vi "Set Default Ref Phase.vi"(8 "error in (no error)":errorcluster, 10 "Default Phase Value (0.0 degrees)":dbl format="%.4f", 11 "VISA resource name":refnum<visa-resource-name>) -> (0 "error out":errorcluster, 3 "VISA resource name out":refnum<visa-resource-name>)   [LabVIEW 2011, in "Fluke 5XXX Series Multicalibrators.lvlib"]
doc: "If two Calibrators are synchronized using 10 MHz IN/OUT, sets the power-up and reset default phase difference between the primary channel on the Calibrator relative to the sync pulse on the 10 MHz IN or OUT terminal.\n\nNote:\n\nThis VI is available only for instrument model 5520A."
uses:
  Fluke 5XXX Series Multicalibrators.lvlib
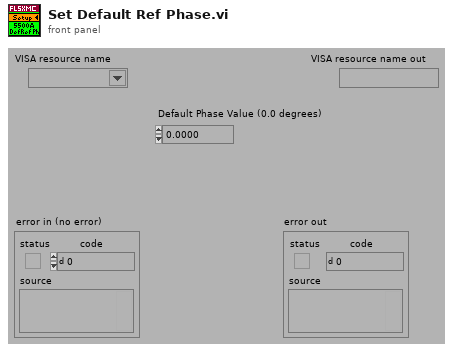
[diagram p1: front panel]
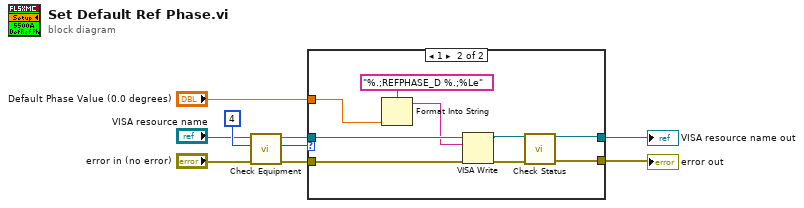
[diagram p0: block diagram]
diagram:
  n1 = call "Check Equipment.vi"("error in (no error)"="error in (no error)", "Bit Mask"=4 ("Numeric"), "VISA resource name"="VISA resource name") -> ("error out"=w9:errorcluster, "Present?"=w8:u32, "VISA resource name out"=w7:refnum<visa-resource-name>)  [unwired: 6 in]
  n2 = case shown="1" w8 {
    tunnel: "Default Phase Value (0.0 degrees)" -> [_ w12]
    tunnel: [w10 w15] -> w1
    tunnel: w9 -> [w11 w20]
    tunnel: w7 -> [w10 w19]
    tunnel: [w11 w18] -> w2
    frame 0, Default {
    }
    frame 1 {
      n3 = Format Into String(format string="%.;REFPHASE_D %.;%Le", w12) -> (resulting string=w13:string)  [unwired: 2 in, 1 out]
      n4 = VISA Write(VISA resource name=w19, write buffer=w13, error in (no error)=w20) -> (VISA resource name out=w16:refnum<visa-resource-name>, error out=w17:errorcluster)  [unwired: 1 out]
      n5 = call "Check Status.vi"("VISA resource name"=w16, "error in (no error)"=w17) -> ("VISA resource name out"=w15:refnum<visa-resource-name>, "error out"=w18:errorcluster)  [unwired: 12 in]
    }
  }
  "VISA resource name out" <- w1
  "error out" <- w2
